vi "Weighted_Mean_fr_NaN_data.vi"(1 "Weighting":dbl[](array[numeric]) format="%.2f", 2 "Data":dbl[](array[numeric]) format="%.4f") -> (0 "Mean value":dbl format="%.2f")   [LabVIEW 2010]
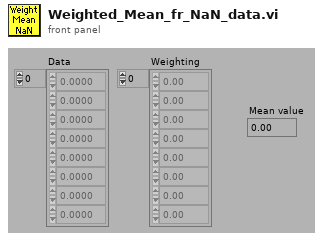
[diagram p1: front panel]
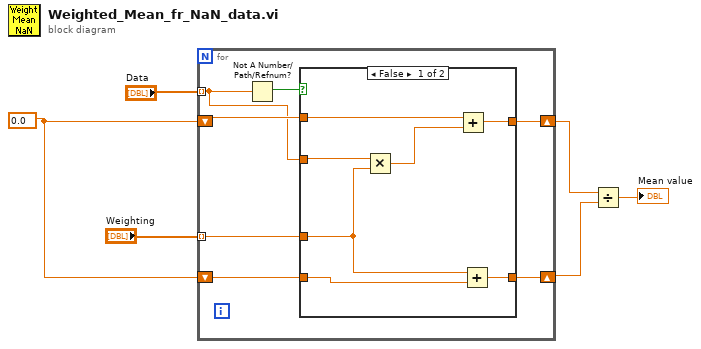
[diagram p0: block diagram]
diagram:
  w4 = 0.0
  n1 = for {
    tunnel: "Data" -> [w10] mode=indexing
    shift-right: [w12] -> w3
    shift-left: w4 -> [w13]
    tunnel: "Weighting" -> [w9] mode=indexing
    shift-right: [w7] -> w2
    shift-left: w4 -> [w8]
    n2 = Not A Number/Path/Refnum?(number/path/refnum=w10) -> (NaN/Path/Refnum?=w11:bool)
    n3 = case shown="False" w11 {
      tunnel: w13 -> [w19 w22]
      tunnel: [w17 w22] -> w12
      tunnel: w10 -> [w20 _]
      tunnel: w9 -> [w16 _]
      tunnel: w8 -> [w15 w21]
      tunnel: [w14 w21] -> w7
      frame False {
        n4 = Multiply(x=w20, y=w16) -> (x*y=w18:dbl)
        n5 = Add(x=w19, y=w18) -> (x+y=w17:dbl)
        n6 = Add(x=w16, y=w15) -> (x+y=w14:dbl)
      }
      frame True {
      }
    }
  }
  n7 = Divide(x=w3, y=w2) -> (x/y=→"Mean value":dbl)
